vi "Configure TS DAC.vi"(8 "error in":errorcluster, 11 "Test Stand in":refnum<class "Generic Test Stand.lvclass">) -> (0 "error out":errorcluster, 3 "Test Stand out":refnum<class "Generic Test Stand.lvclass">)   [LabVIEW 2019, in "Generic Test Stand.lvclass"]
uses:
  Generic Test Stand.lvclass
  Generic Test Stand.lvclass/Generic Test Stand.ctl
  DAC/DAC.lvclass
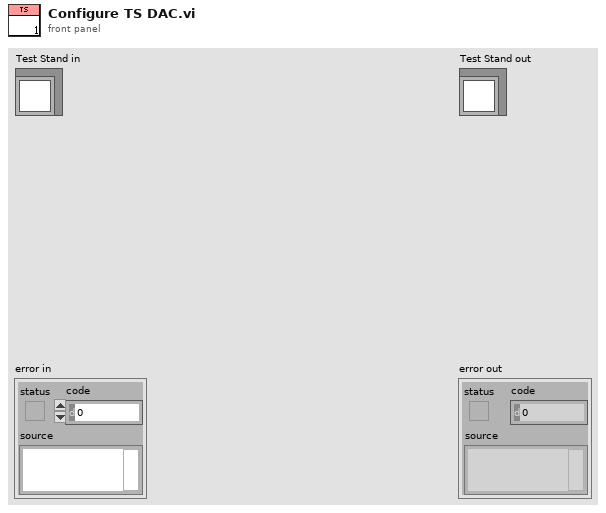
[diagram p1: front panel]
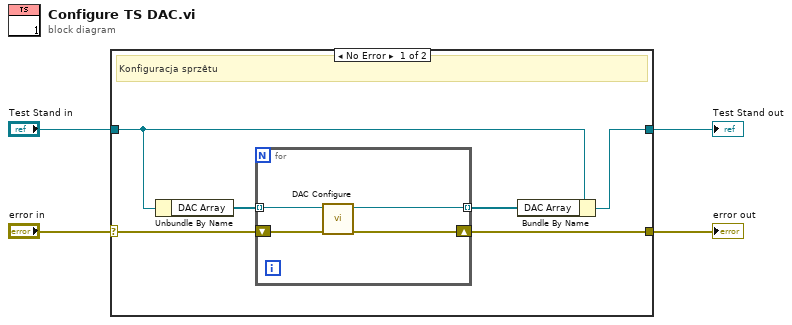
[diagram p0: block diagram]
diagram:
  n1 = case shown="No Error" "error in" {
    selector: "error in" -> [w10 w16]
    tunnel: "Test Stand in" -> [w6 w15]
    tunnel: [w5 w15] -> w2
    tunnel: [w9 w16] -> w1
    frame No Error {
      # "Konfiguracja sprzêtu"
      n2 = Unbundle By Name(w6) -> ("DAC Array"=w8:refnum<class "DAC.lvclass">[])
      n3 = for {
        tunnel: w8 -> [w14] mode=indexing
        tunnel: [w13] -> w7 mode=indexing
        shift-right: [w12] -> w9
        shift-left: w10 -> [w11]
        n4 = call-dynamic "DAC Configure.vi"("error in (no error)"=w11, "DAC in"=w14) -> ("error out"=w12:errorcluster, "DAC out"=w13:refnum<class "DAC.lvclass">)  [unwired: 8 in]
      }
      n5 = Bundle By Name(cluster=w6, "DAC Array"=w7) -> (w5:refnum<class "Generic Test Stand.lvclass">)
    }
    frame Error {
    }
  }
  "error out" <- w1
  "Test Stand out" <- w2
